vi "TL-TEC_Init-2.vi"(0 "ThorLabsPro8000":refnum<visa-resource-name>, 5 "ThorLabsCluster":T1) -> (15 "Error Out":errorcluster)   [LabVIEW 2012]
uses:
  ThorLabsCluster.ctl
panel:
  out "On Line Mode\n0=CP 1=CC":dbl
  out "On Line Limit (mA)":dbl
  out "On Line Polarity\n0=AG 1=CG":dbl
  out "On Line TP":dbl
  out "On Line TP Slot":dbl
  out "On Line Current (mA)":dbl
  out "On Line LD Slot":dbl
  out "Off Line Mode\n0=CP 1=CC":dbl
  out "Off Line Limit (mA)":dbl
  out "Off Line Polarity\n0=AG 1=CG":dbl
  out "Off Line TP":dbl
  out "Off Line TP Slot":dbl
  out "Off Line Current (mA)":dbl
  out "Off Line LD Slot":dbl
  out "WarmUpTime":dbl
  out "TSOA Temp (C)":dbl
  out "TSOA TempSens\n0=AD 1=THL":dbl
  out "TSOA Twin":dbl
  out "TSOA D-Const":dbl
  out "TSOA I-Const":dbl
  out "TSOA P-Const":dbl
  out "TSOA TEC Slot":dbl
  out "Etalon Temp (C)":dbl
  out "Etalon TempSens\n0=AD 1=THL":dbl
  out "Etalon Twin":dbl
  out "Etalon D-Const":dbl
  out "Etalon I-Const":dbl
  out "Etalon P-Const":dbl
  out "Etalon TEC Slot":dbl
  out "Off Line Temp (C)":dbl
  out "Off Line TempSens\n0=AD 1=THL":dbl
  out "Off Line Twin (C)":dbl
  out "Off Line D-Const":dbl
  out "Off Line I-Const":dbl
  out "Off Line P-Const":dbl
  out "Off Line TEC Slot":dbl
  out "On Line Temp (C)":dbl
  out "On Line TempSens\n0=AD 1=THL":dbl
  out "On Line Twin (C)":dbl
  out "On Line D-Const":dbl
  out "On Line I-Const":dbl
  out "On Line P-Const":dbl
  out "On Line TEC Slot":dbl
  out "LD Strings":string[](array[string])
  out "TEC Strings":string[](array[string])
  out "ID String":string
  out "VISA Out":string
  # "Thorlabs Pro 8000"
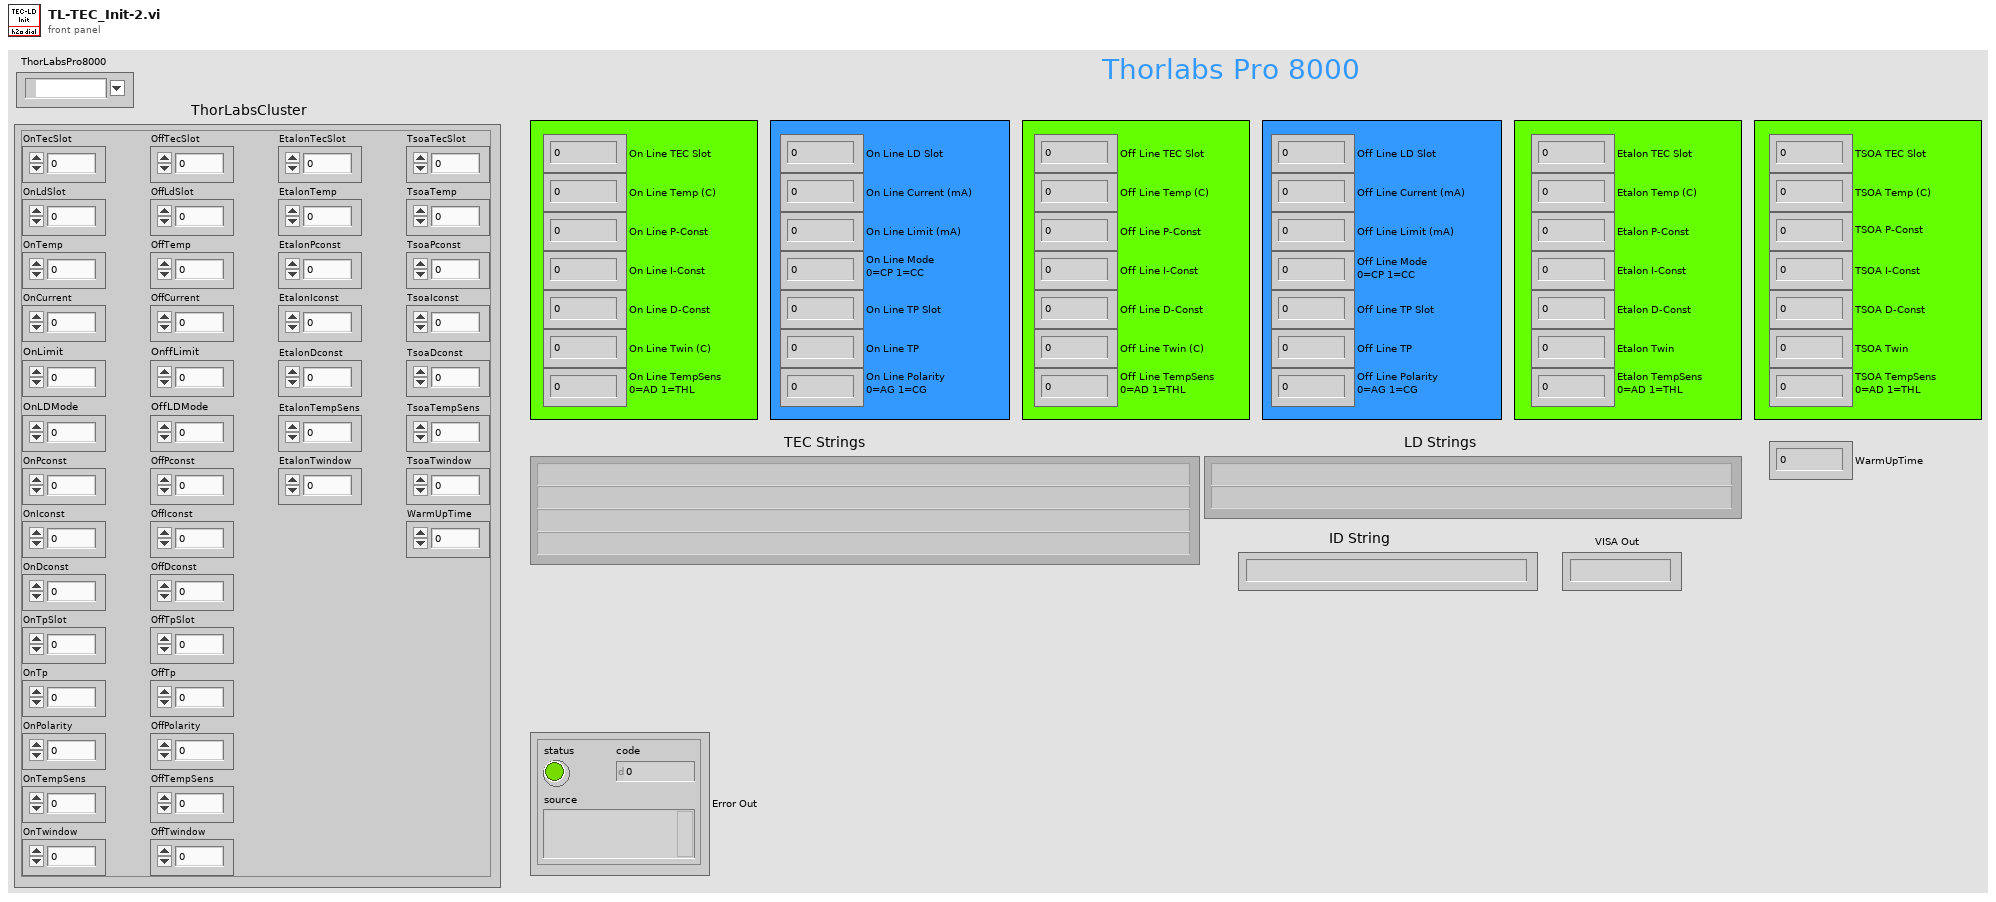
[diagram p1: front panel]
types:
  T1 = typedef "ThorLabsCluster.ctl" = cluster{"OnTecSlot":dbl, "OnLdSlot":dbl, "OnTemp":dbl, "OnCurrent":dbl, "OnPconst":dbl, "OnIconst":dbl, "OnDconst":dbl, "OnTpSlot":dbl, "OnTp":dbl, "OnPolarity":dbl, "OnTempSens":dbl, "OnTwindow":dbl, "OffTecSlot":dbl, "OffLdSlot":dbl, "OffTemp":dbl, "OffCurrent":dbl, "OffPconst":dbl, "OffIconst":dbl, "OffDconst":dbl, "OffTpSlot":dbl, "OffTp":dbl, "OffPolarity":dbl, "OffTempSens":dbl, "OffTwindow":dbl, "EtalonTecSlot":dbl, "EtalonTemp":dbl, "EtalonPconst":dbl, "EtalonIconst":dbl, "EtalonDconst":dbl, "EtalonTempSens":dbl, "EtalonTwindow":dbl, "TsoaTecSlot":dbl, "TsoaTemp":dbl, "TsoaPconst":dbl, "TsoaIconst":dbl, "TsoaDconst":dbl, "TsoaTempSens":dbl, "TsoaTwindow":dbl, "WarmUpTime":dbl, "OnLimit":dbl, "OnffLimit":dbl, "OnLDMode":dbl, "OffLDMode":dbl}
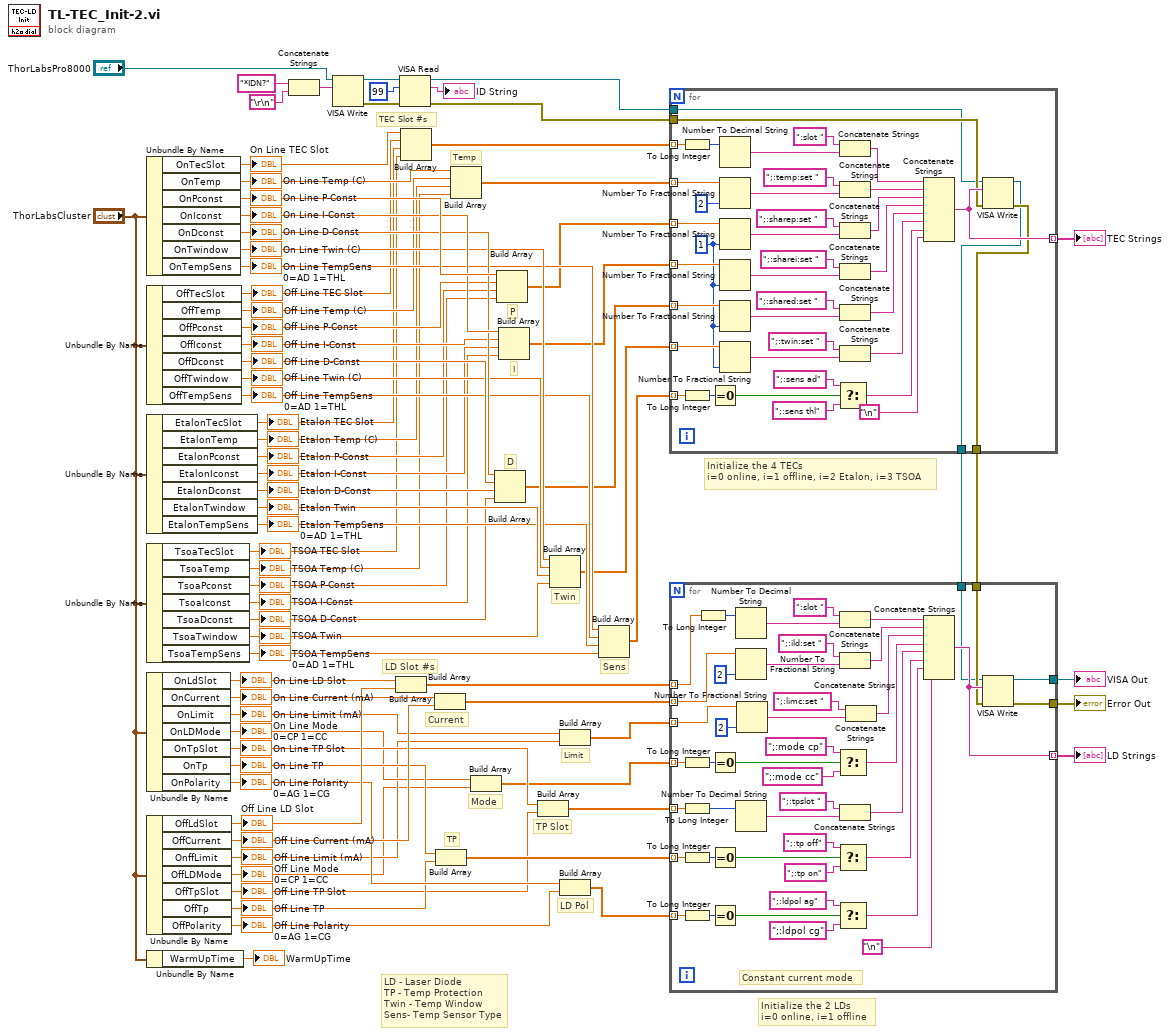
[diagram p0: block diagram]
diagram:
  # "Mode"
  # "Limit"
  # "LD - Laser Diode\nTP - Temp Protection\nTwin - Temp Window\nSens- Temp Sensor Type"
  # "Initialize the 2 LDs\ni=0 online, i=1 offline"
  # "LD Slot #s"
  # "Current"
  # "TP Slot"
  # "TP"
  # "LD Pol"
  # "Initialize the 4 TECs\ni=0 online, i=1 offline, i=2 Etalon, i=3 TSOA"
  # "Sens"
  # "Twin"
  # "D"
  # "I"
  # "P"
  # "Temp"
  # "TEC Slot #s"
  n1 = Unbundle By Name("ThorLabsCluster") -> ("OnTecSlot"=w74:dbl, "OnTemp"=w73:dbl, "OnPconst"=w72:dbl, "OnIconst"=w71:dbl, "OnDconst"=w70:dbl, "OnTwindow"=w69:dbl, "OnTempSens"=w68:dbl)
  "On Line TEC Slot" <- w74
  "On Line P-Const" <- w72
  "On Line I-Const" <- w71
  "On Line D-Const" <- w70
  "On Line Twin (C)" <- w69
  "On Line TempSens\n0=AD 1=THL" <- w68
  "On Line Temp (C)" <- w73
  n2 = Unbundle By Name("ThorLabsCluster") -> ("OffTecSlot"=w67:dbl, "OffTemp"=w66:dbl, "OffPconst"=w65:dbl, "OffIconst"=w64:dbl, "OffDconst"=w63:dbl, "OffTwindow"=w62:dbl, "OffTempSens"=w61:dbl)
  "Off Line TEC Slot" <- w67
  "Off Line P-Const" <- w65
  "Off Line I-Const" <- w64
  "Off Line D-Const" <- w63
  "Off Line Twin (C)" <- w62
  "Off Line TempSens\n0=AD 1=THL" <- w61
  "Off Line Temp (C)" <- w66
  n3 = Unbundle By Name("ThorLabsCluster") -> ("EtalonTecSlot"=w60:dbl, "EtalonTemp"=w59:dbl, "EtalonPconst"=w58:dbl, "EtalonIconst"=w57:dbl, "EtalonDconst"=w56:dbl, "EtalonTwindow"=w55:dbl, "EtalonTempSens"=w54:dbl)
  "Etalon TEC Slot" <- w60
  "Etalon P-Const" <- w58
  "Etalon I-Const" <- w57
  "Etalon D-Const" <- w56
  "Etalon Twin" <- w55
  "Etalon TempSens\n0=AD 1=THL" <- w54
  "Etalon Temp (C)" <- w59
  n4 = Unbundle By Name("ThorLabsCluster") -> ("TsoaTecSlot"=w53:dbl, "TsoaTemp"=w52:dbl, "TsoaPconst"=w51:dbl, "TsoaIconst"=w50:dbl, "TsoaDconst"=w49:dbl, "TsoaTwindow"=w48:dbl, "TsoaTempSens"=w47:dbl)
  "TSOA TEC Slot" <- w53
  "TSOA P-Const" <- w51
  "TSOA I-Const" <- w50
  "TSOA D-Const" <- w49
  "TSOA Twin" <- w48
  "TSOA TempSens\n0=AD 1=THL" <- w47
  "TSOA Temp (C)" <- w52
  n5 = Unbundle By Name("ThorLabsCluster") -> ("OnLdSlot"=w29:dbl, "OnCurrent"=w27:dbl, "OnLimit"=w4:dbl, "OnLDMode"=w3:dbl, "OnTpSlot"=w10:dbl, "OnTp"=w11:dbl, "OnPolarity"=w12:dbl)
  "On Line LD Slot" <- w29
  "On Line Current (mA)" <- w27
  "On Line TP Slot" <- w10
  "On Line TP" <- w11
  "On Line Polarity\n0=AG 1=CG" <- w12
  "On Line Limit (mA)" <- w4
  "On Line Mode\n0=CP 1=CC" <- w3
  n6 = Unbundle By Name("ThorLabsCluster") -> ("OffLdSlot"=w28:dbl, "OffCurrent"=w26:dbl, "OnffLimit"=w2:dbl, "OffLDMode"=w1:dbl, "OffTpSlot"=w7:dbl, "OffTp"=w8:dbl, "OffPolarity"=w9:dbl)
  "Off Line LD Slot" <- w28
  "Off Line Current (mA)" <- w26
  "Off Line TP Slot" <- w7
  "Off Line TP" <- w8
  "Off Line Polarity\n0=AG 1=CG" <- w9
  "Off Line Limit (mA)" <- w2
  "Off Line Mode\n0=CP 1=CC" <- w1
  n7 = Unbundle By Name("ThorLabsCluster") -> ("WarmUpTime"=→"WarmUpTime":dbl)
  n8 = Concatenate Strings("*IDN?" ("string"), "\r\n") -> (w38:string)
  n9 = VISA Write(VISA resource name="ThorLabsPro8000", write buffer=w38) -> (VISA resource name out=w36:refnum<visa-resource-name>, error out=w32:errorcluster)  [unwired: 1 in, 1 out]
  n10 = Build Array(w29, w28) -> (w25:dbl[])
  n11 = VISA Read(VISA resource name=w36, byte count=u32 99, error in (no error)=w32) -> (VISA resource name out=w35:refnum<visa-resource-name>, read buffer=→"ID String":string, error out=w31:errorcluster)  [unwired: 1 out]
  n12 = Build Array(w74, w67, w60, w53) -> (w46:dbl[])
  n13 = Build Array(w27, w26) -> (w24:dbl[])
  n14 = Build Array(w11, w8) -> (w22:dbl[])
  n15 = Build Array(w73, w66, w59, w52) -> (w45:dbl[])
  n16 = Build Array(w3, w1) -> (w5:dbl[])
  n17 = Build Array(w70, w63, w56, w49) -> (w42:dbl[])
  n18 = Build Array(w72, w65, w58, w51) -> (w44:dbl[])
  n19 = Build Array(w71, w64, w57, w50) -> (w41:dbl[])
  n20 = Build Array(w10, w7) -> (w23:dbl[])
  n21 = Build Array(w69, w62, w55, w48) -> (w40:dbl[])
  n22 = Build Array(w4, w2) -> (w6:dbl[])
  n23 = Build Array(w12, w9) -> (w21:dbl[])
  n24 = Build Array(w68, w61, w54, w47) -> (w43:dbl[])
  n25 = for {
    tunnel: w46 -> [w113] mode=indexing
    tunnel: w45 -> [w111] mode=indexing
    tunnel: w44 -> [w92] mode=indexing
    tunnel: w43 -> [w110] mode=indexing
    tunnel: w42 -> [w91] mode=indexing
    tunnel: w41 -> [w90] mode=indexing
    tunnel: w40 -> [w89] mode=indexing
    tunnel: w35 -> [w78]
    tunnel: w31 -> [w79]
    tunnel: [w80] -> w20 mode=indexing
    tunnel: [w76] -> w18
    tunnel: [w75] -> w17
    w77 = i16 1 ("precision (6)")
    n26 = To Long Integer(number=w113) -> (32bit integer=w112:i32)
    n27 = To Long Integer(number=w110) -> (32bit integer=w97:i32)
    n28 = Equal To 0?(x=w97) -> (x = 0?=w94:bool)
    n29 = Number To Decimal String(number=w112) -> (decimal integer string=w109:string)  [unwired: 1 in]
    n30 = Number To Fractional String(number=w111, precision (6)=i16 2) -> (F-format string=w107:string)  [unwired: 2 in]
    n31 = Number To Fractional String(number=w92, precision (6)=w77) -> (F-format string=w102:string)  [unwired: 2 in]
    n32 = Number To Fractional String(number=w90, precision (6)=w77) -> (F-format string=w101:string)  [unwired: 2 in]
    n33 = Number To Fractional String(number=w91, precision (6)=w77) -> (F-format string=w100:string)  [unwired: 2 in]
    n34 = Number To Fractional String(number=w89, precision (6)=w77) -> (F-format string=w99:string)  [unwired: 2 in]
    n35 = Select(t=";:sens ad" ("string"), s=w94, f=";:sens thl" ("string")) -> (s? t:f=w84:string)
    n36 = Concatenate Strings(":slot ", w109) -> (w81:string)
    n37 = Concatenate Strings(";:temp:set " ("write buffer"), w107) -> (w93:string)
    n38 = Concatenate Strings(";:sharep:set " ("write buffer"), w102) -> (w88:string)
    n39 = Concatenate Strings(";:sharei:set " ("write buffer"), w101) -> (w87:string)
    n40 = Concatenate Strings(";:shared:set " ("write buffer"), w100) -> (w86:string)
    n41 = Concatenate Strings(";:twin:set " ("write buffer"), w99) -> (w85:string)
    n42 = Concatenate Strings(w81, w93, w88, w87, w86, w85, w84, "\n") -> (w80:string)
    n43 = VISA Write(VISA resource name=w78, write buffer=w80, error in (no error)=w79) -> (VISA resource name out=w75:refnum<visa-resource-name>, error out=w76:errorcluster)  [unwired: 1 out]
  }
  "TEC Strings" <- w20
  n44 = for {
    tunnel: w25 -> [w157] mode=indexing
    tunnel: w24 -> [w154] mode=indexing
    tunnel: w23 -> [w153] mode=indexing
    tunnel: w22 -> [w152] mode=indexing
    tunnel: w21 -> [w156] mode=indexing
    tunnel: [w133] -> w19 mode=indexing
    tunnel: w18 -> [w132]
    tunnel: w17 -> [w131]
    tunnel: [w130] -> w16
    tunnel: [w129] -> w15
    tunnel: w6 -> [w126] mode=indexing
    tunnel: w5 -> [w122] mode=indexing
    # "Constant current mode"
    n45 = To Long Integer(number=w122) -> (32bit integer=w123:i32)
    n46 = To Long Integer(number=w153) -> (32bit integer=w142:i32)
    n47 = To Long Integer(number=w152) -> (32bit integer=w151:i32)
    n48 = To Long Integer(number=w156) -> (32bit integer=w150:i32)
    n49 = To Long Integer(number=w157) -> (32bit integer=w155:i32)
    n50 = Equal To 0?(x=w123) -> (x = 0?=w118:bool)
    n51 = Equal To 0?(x=w151) -> (x = 0?=w144:bool)
    n52 = Equal To 0?(x=w150) -> (x = 0?=w143:bool)
    n53 = Number To Decimal String(number=w155) -> (decimal integer string=w148:string)  [unwired: 1 in]
    n54 = Number To Fractional String(number=w154, precision (6)=i16 2) -> (F-format string=w147:string)  [unwired: 2 in]
    n55 = Number To Decimal String(number=w142) -> (decimal integer string=w141:string)  [unwired: 1 in]
    n56 = Number To Fractional String(number=w126, precision (6)=i16 2) -> (F-format string=w128:string)  [unwired: 2 in]
    n57 = Select(t=";:mode cp" ("write buffer"), s=w118, f=";:mode cc" ("write buffer")) -> (s? t:f=w115:string)
    n58 = Select(t=";:tp off" ("write buffer"), s=w144, f=";:tp on" ("write buffer")) -> (s? t:f=w120:string)
    n59 = Select(t=";:ldpol ag" ("write buffer"), s=w143, f=";:ldpol cg" ("write buffer")) -> (s? t:f=w119:string)
    n60 = Concatenate Strings(":slot ", w148) -> (w136:string)
    n61 = Concatenate Strings(";:ild:set " ("write buffer"), w147) -> (w135:string)
    n62 = Concatenate Strings(";:tpslot " ("write buffer"), w141) -> (w121:string)
    n63 = Concatenate Strings(";:limc:set " ("write buffer"), w128) -> (w124:string)
    n64 = Concatenate Strings(w136, w135, w124, w115, w121, w120, w119, "\n") -> (w133:string)
    n65 = VISA Write(VISA resource name=w131, write buffer=w133, error in (no error)=w132) -> (VISA resource name out=w130:refnum<visa-resource-name>, error out=w129:errorcluster)  [unwired: 1 out]
  }
  "VISA Out" <- w16
  "Error Out" <- w15
  "LD Strings" <- w19
